vi "关闭基恩士PLC连接.vi"(8 "错误输入（无错误）":errorcluster, 11 "Keyence ID":refnum<k5>) -> (0 "错误输出":errorcluster)   [LabVIEW 2017]
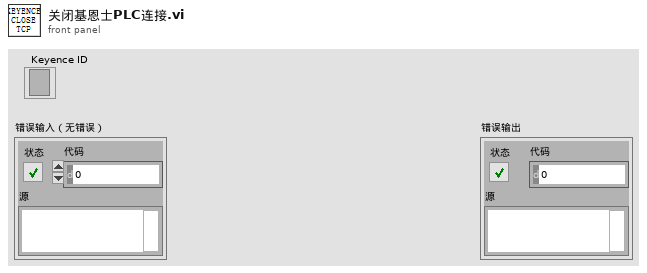
[diagram p1: front panel]
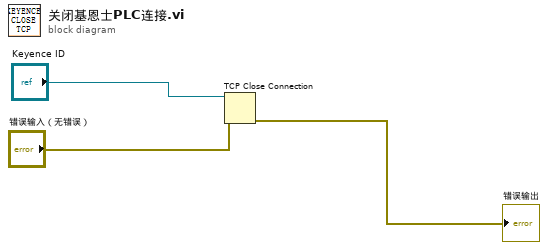
[diagram p0: block diagram]
diagram:
  n1 = TCP Close Connection(connection ID="Keyence ID", error in (no error)="错误输入（无错误）") -> (error out=→"错误输出":errorcluster)  [unwired: 1 in, 1 out]
